vi "thermocoupleSub.vi"(8 "Below 0?":bool, 11 "Voltage(mV)":dbl) -> (3 "output variable":dbl)   [LabVIEW 2023]
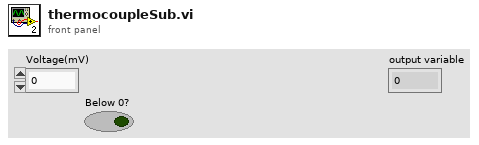
[diagram p1: front panel]
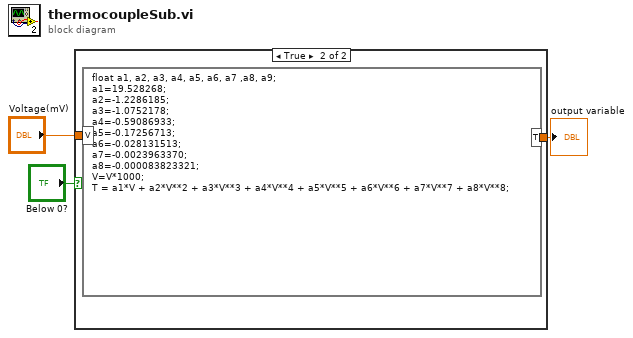
[diagram p0: block diagram]
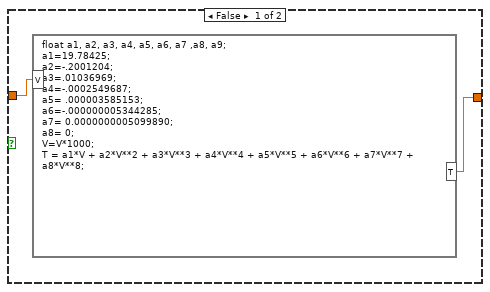
[diagram p2: hidden frame]
diagram:
  n1 = case shown="True" "Below 0?" {
    tunnel: "Voltage(mV)" -> [w5 w7]
    tunnel: [w4 w6] -> w2
    frame False {
      n2 = formula code="float a1, a2, a3, a4, a5, a6, a7 ,a8, a9;\na1=19.78425;\na2=-.2001204;\na3=.01036969;\na4=-.0002549687;\na5= .000003585153;\na6=-.000000005344285;\na7= 0.0000000005099890;\na8= 0;\nV=V*1000;\nT = a1*V + a2*V**2 + a3*V**3 + a4*V**4 + a5*V**5 + a6*V**6 + a7*V**7 + a8*V**8;"("V"=w5) -> ("T"=w4:dbl)
    }
    frame True {
      n3 = formula code="float a1, a2, a3, a4, a5, a6, a7 ,a8, a9;\na1=19.528268;\na2=-1.2286185;\na3=-1.0752178;\na4=-0.59086933;\na5=-0.17256713;\na6=-0.028131513;\na7=-0.0023963370;\na8=-0.000083823321;\nV=V*1000;\nT = a1*V + a2*V**2 + a3*V**3 + a4*V**4 + a5*V**5 + a6*V**6 + a7*V**7 + a8*V**8;"("V"=w7) -> ("T"=w6:dbl)
    }
  }
  "output variable" <- w2
